vi "testdata.vi"(0 "温度":sgl format="%#_13g", 1 "时间":timestamp, 2 "error IO":errorcluster, 5 "uid":i16, 7 "纬度":sgl format="%#_13g", 9 "经度":sgl format="%#_13g", 11 "滑动杆":i16(slide) scale=3.5..18.0, 12 "地图":refnum<k7>(container) caption="网页浏览器") -> (3 "储运信息簇":T1 {"记录时间" format="%<%H:%M:%S\n%Y/%m/%d>T"}, 4 "定位":bool, 6 "温度":sgl, 8 "uid":i16, 10 "纬度显示":string, 13 "错误输出":errorcluster, 15 "经度显示":string)   [LabVIEW 2018]
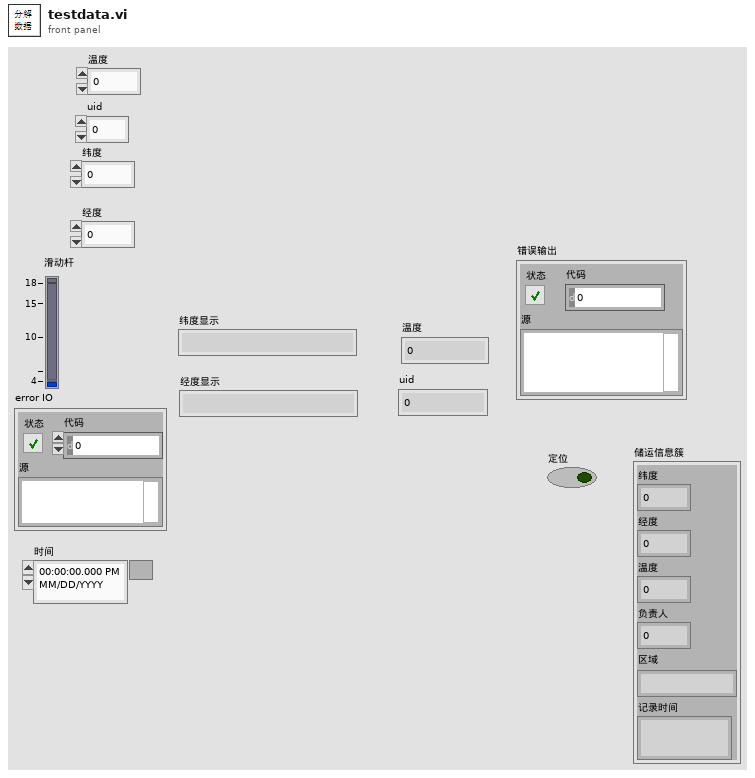
[diagram p1: front panel]
types:
  T1 = typedef "储运信息.ctl" = cluster{"纬度":sgl, "经度":sgl, "温度":sgl, "负责人":i32, "区域":string, "记录时间":timestamp}
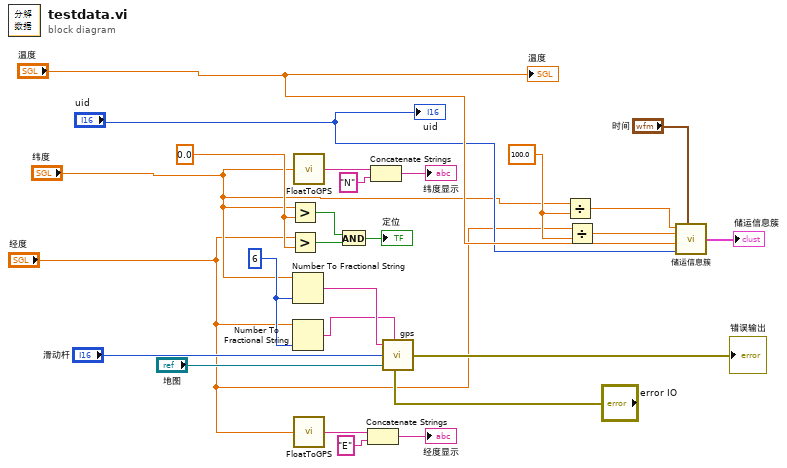
[diagram p0: block diagram]
diagram:
  w5 = 100.0
  w19 = i16 6 ("精度(6)")
  w26 = 0.0 ("y")
  n1 = Greater?(x="纬度", y=w26) -> (0:w23:bool)
  n2 = Greater?(x="经度", y=w26) -> (0:w24:bool)
  n3 = Number To Fractional String(number="纬度", precision (6)=w19) -> (F-format string=w13:string)  [unwired: 2 in]
  n4 = Number To Fractional String(number="经度", precision (6)=w19) -> (F-format string=w12:string)  [unwired: 2 in]
  n5 = call "FloatToGPS.vi"("数字"="纬度") -> ("string"=w20:string)
  n6 = call "FloatToGPS.vi"("数字"="经度") -> ("string"=w18:string)
  n7 = And(x=w23, y=w24) -> (x .and. y?=→"定位":bool)
  n8 = Concatenate Strings(w18, "E" ("字符串")) -> (→"经度显示":string)
  n9 = Concatenate Strings(w20, "N" ("字符串")) -> (→"纬度显示":string)
  n10 = call "gps.vi"("纬度"=w13, "经度"=w12, "滑动杆"="滑动杆", "地图"="地图", "error IO"="error IO") -> ("错误输出"=→"错误输出":errorcluster)
  n11 = Divide(x="纬度", y=w5) -> (x/y=w7:dbl)
  n12 = Divide(x="经度", y=w5) -> (x/y=w6:dbl)
  n13 = call "储运信息簇.vi"("纬度"=w7, "经度"=w6, "温度"="温度", "编号"="uid", "时间"="时间") -> ("待写入的簇"=→"储运信息簇":T1)
  "温度" <- "温度"
  "uid" <- "uid"
